vi "DQMH-GenNet Return DQMH Queue if GenNet Queue is invalid.vi"(7 "Message Queue in":refnum<class "Delacor_lib_QMH_Message Queue.lvclass">, 8 "error in (no error)":errorcluster, 11 "DQMH-GenNet Message Queue in":refnum<class "DQMH-GenNet Message Queue.lvclass">) -> (0 "error out":errorcluster, 3 "Message Queue out":refnum<class "Delacor_lib_QMH_Message Queue.lvclass">)   [LabVIEW 2020, in "hse-gennet.lvlib" / "DQMH-GenNet Message Queue.lvclass"]
doc: "____\nHAMPEL SOFTWARE ENGINEERING v3.8.0 (2023-12-18 14:41)"
uses:
  DQMH-GenNet Message Queue.lvclass
  C:/Program Files (x86)/National Instruments/LabVIEW 2020/vi.lib/Delacor/Delacor QMH/Libraries/Message Queue_class/Delacor_lib_QMH_Message Queue.lvclass
  <vilib>/Delacor/Delacor QMH/Libraries/Message Queue_class/Delacor_lib_QMH_Message Queue.lvclass
  <vilib>/Delacor/Delacor QMH/Libraries/Message Queue_class/Delacor_lib_QMH_Message Queue.lvclass/Delacor_lib_QMH_Message Queue.ctl
  <vilib>/Delacor/Delacor QMH/Libraries/Message Queue_class/Delacor_lib_QMH_Get Message Queue.vi
  DQMH-GenNet Message Queue.lvclass/DQMH-GenNet Message Queue.ctl
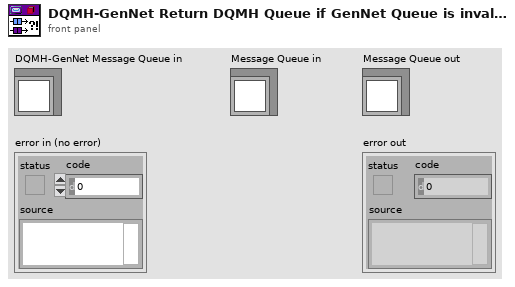
[diagram p1: front panel]
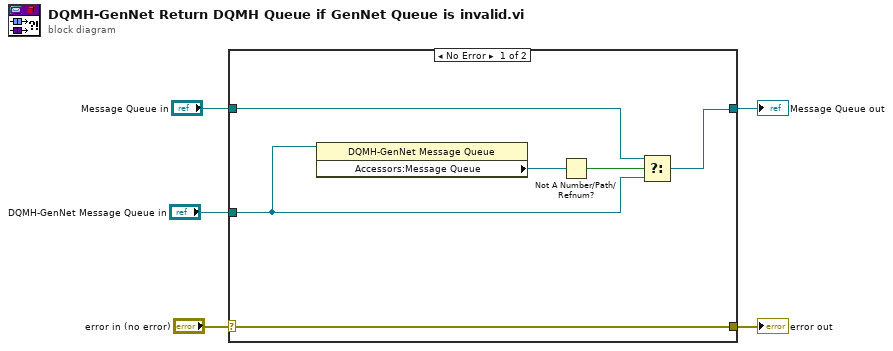
[diagram p0: block diagram]
diagram:
  n1 = case shown="No Error" "error in (no error)" {
    selector: "error in (no error)" -> [w11 w13]
    tunnel: [w11 w13] -> w4
    tunnel: [w9 w12] -> w2
    tunnel: "DQMH-GenNet Message Queue in" -> [w8 _]
    tunnel: "Message Queue in" -> [w10 w12]
    frame No Error {
      n2 = property class="DQMH-GenNet Message Queue"(reference=w8) -> ("Accessors:Message Queue"=w7:refnum<queue>)  [unwired: 1 in, 2 out]
      n3 = Not A Number/Path/Refnum?(number/path/refnum=w7) -> (NaN/Path/Refnum?=w6:bool)
      n4 = Select(t=w10, s=w6, f=w8) -> (s? t:f=w9:refnum<class "Delacor_lib_QMH_Message Queue.lvclass">)
    }
    frame Error {
    }
  }
  "error out" <- w4
  "Message Queue out" <- w2
